vi "FITS Profile Execution Time.vi"() -> ()   [LabVIEW 2024]
uses:
  FITS cluster Header Row.ctl
  FITS enum Data Type.ctl
  b220779a-bb3b-4bf7-b569-9287463a0bc4.vi
  bbd996fc-5987-4dd4-a412-da4c3bdc7f49.vi
  c6e7a5a2-5daf-4f44-8c18-a00dc3bdbb1d.vi
  bac9f9f0-713b-42df-8ddf-044b6a61410f.vi
  4b24a88b-7104-40e5-83d7-27edd1db6c6a.vi
  gfitsio/gfitsio-write-key-integer.vi
  gfitsio/gfitsio-write-key-string.vi
  gfitsio/gfitsio-write-key-double.vi
  gfitsio/gfitsio.lvlib
panel:
  out "x-y":u32
  in  "error in (no error)":errorcluster
  out "FITS Hdr Rows":T1[](array[typedef])
  out "elapsed time":u32
  out "hdr writes":u32[](array[numeric])
  out "open":u32
  out "error out":errorcluster
  in  "file path (dialog if empty)":path
  in  "FITS Template":path=path "C:/Users/gsfcprime/Documents/LabVIEW Data/FITS Templates/header0.json"
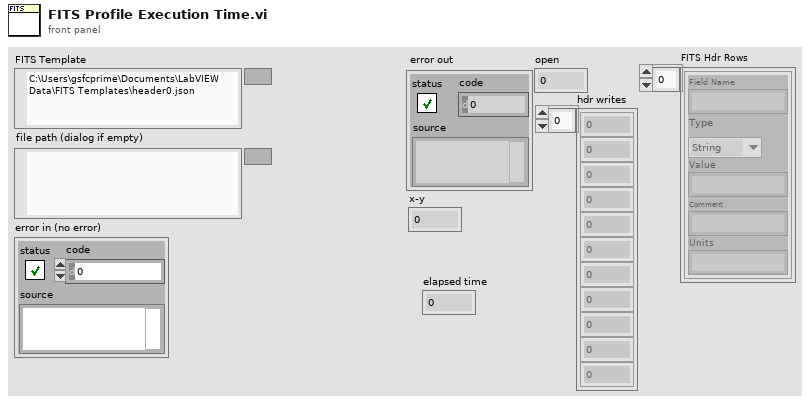
[diagram p1: front panel]
types:
  T1 = typedef "FITS cluster Header Row.ctl" = cluster{"Field Name":string, "Type":T2, "Value":string, "Comment":string, "Units":string}
  T2 = typedef "FITS enum Data Type.ctl" = enum16{"String", "Integer", "Float"}
  T3 = typedef "gfitsio.lvlib/gfitsio-refnum.ctl" = u64
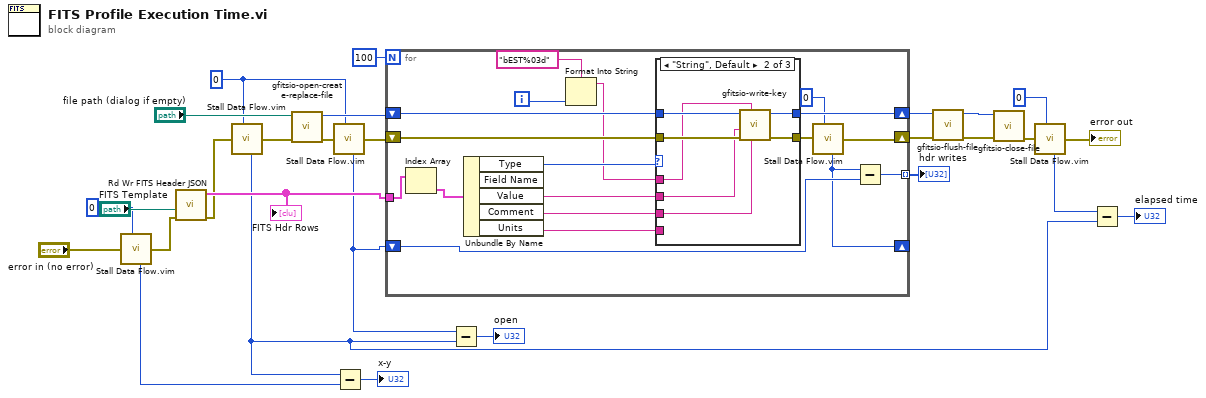
[diagram p0: block diagram]
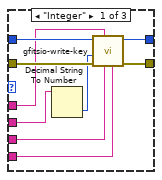
[diagram p2: hidden frame]
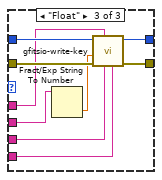
[diagram p3: hidden frame]
diagram:
  w21 = u32 0 ("milliseconds to wait")
  n1 = call "Stall Data Flow.vim"("value in"="error in (no error)", "milliseconds to wait"=u32 0) -> ("millisecond timer value"=w2:u32, "value out"=w5:errorcluster)
  n2 = call "Rd Wr FITS Header JSON.vi"("error in (no error)"=w5, "FITS Template"="FITS Template") -> ("error out"=w23:errorcluster, "FITS Hdr Rows"=w25:T1[])  [unwired: 8 in]
  "FITS Hdr Rows" <- w25
  n3 = call "Stall Data Flow.vim"("value in"=w23, "milliseconds to wait"=w21) -> ("millisecond timer value"=w3:u32, "value out"=w24:errorcluster)
  n4 = call "gfitsio-open-create-replace-file.vi"("error in (no error)"=w24, "file path (dialog if empty)"="file path (dialog if empty)") -> ("error out"=w22:errorcluster, "gfits refnum"=w26:T3)  [unwired: 7 in, 1 out]
  n5 = call "Stall Data Flow.vim"("value in"=w22, "milliseconds to wait"=w21) -> ("millisecond timer value"=w14:u32, "value out"=w20:errorcluster)
  n6 = Subtract(x=w3, y=w2) -> (x-y=→"x-y":u32)
  n7 = for {
    N: 100 -> [_]
    shift-right: [w44] -> w10
    shift-left: w26 -> [w46]
    shift-right: [w38] -> w11
    shift-left: w20 -> [w45]
    tunnel: w25 -> [w33]
    tunnel: [w36] -> w13 mode=indexing
    shift-right: [w34] -> _
    shift-left: w14 -> [w35]
    i -> [w30]
    n8 = Index Array(array=w33) -> (element=w32:T1)  [unwired: 1 in]
    n9 = Unbundle By Name(w32) -> ("Type"=w43:T2, "Value"=w41:string, "Comment"=w42:string, "Units"=w40:string)  [unwired: 1 out]
    n10 = Format Into String(format string="bEST%03d", w30) -> (resulting string=w29:string)  [unwired: 2 in, 1 out]
    n11 = case shown="\"String\", Default" w43 {
      tunnel: w46 -> [w55 w62 w71]
      tunnel: w45 -> [w54 w61 w70]
      tunnel: [w53 w60 w69] -> w44
      tunnel: [w52 w59 w68] -> w39
      tunnel: w29 -> [w51 w58 w67]
      tunnel: w42 -> [w50 w57 w66]
      tunnel: w41 -> [w49 w56 w65]
      tunnel: w40 -> [w47 _ w63]
      frame "Integer" {
        n12 = Decimal String To Number(string=w49) -> (number=w48:i32)  [unwired: 2 in, 1 out]
        n13 = call-poly "gfitsio-write-key.vi"("units"=w47, "comment"=w50, "keyname"=w51, "error in (no error)"=w54, "value"=w48, "gfits refnum"=w55) -> ("error out"=w52:errorcluster, "dup gfits refnum"=w53:T3)  [unwired: 4 in]
      }
      frame "String", Default {
        n14 = call-poly "gfitsio-write-key.vi"("comment"=w57, "keyname"=w58, "error in (no error)"=w61, "value"=w56, "gfits refnum"=w62) -> ("error out"=w59:errorcluster, "dup gfits refnum"=w60:T3)  [unwired: 5 in]
      }
      frame "Float" {
        n15 = Fract/Exp String To Number(string=w65) -> (number=w64:dbl)  [unwired: 3 in, 1 out]
        n16 = call-poly "gfitsio-write-key.vi"("units"=w63, "comment"=w66, "keyname"=w67, "error in (no error)"=w70, "value"=w64, "gfits refnum"=w71) -> ("error out"=w68:errorcluster, "dup gfits refnum"=w69:T3)  [unwired: 4 in]
      }
    }
    n17 = call "Stall Data Flow.vim"("value in"=w39, "milliseconds to wait"=u32 0) -> ("millisecond timer value"=w34:u32, "value out"=w38:errorcluster)
    n18 = Subtract(x=w34, y=w35) -> (x-y=w36:u32)
  }
  "hdr writes" <- w13
  n19 = Subtract(x=w14, y=w3) -> (x-y=→"open":u32)
  n20 = call "gfitsio-flush-file.vi"("error in (no error)"=w11, "gfits refnum"=w10) -> ("error out"=w8:errorcluster, "dup gfits refnum"=w9:T3)  [unwired: 8 in]
  n21 = call "gfitsio-close-file.vi"("error in (no error)"=w8, "gfits refnum"=w9) -> ("error out"=w19:errorcluster)  [unwired: 8 in, 1 out]
  n22 = call "Stall Data Flow.vim"("value in"=w19, "milliseconds to wait"=u32 0) -> ("millisecond timer value"=w16:u32, "value out"=→"error out":errorcluster)
  n23 = Subtract(x=w16, y=w3) -> (x-y=→"elapsed time":u32)
